vi "Oracle Popup.vi"(8 "error in":errorcluster, 11 "SR List in":T1[](array[typedef]) {"Last Updated" format="%<%x>T"}) -> (0 "error out":errorcluster, 1 "New SRs?":bool, 3 "SR List out":T1[](array[typedef]) {"Last Updated" format="%<%x>T"})   [LabVIEW 2018]
uses:
  SR Cluster.ctl
  <vilib>/Utility/miscctls.llb/LVPointTypeDef.ctl
  <vilib>/Utility/miscctls.llb/LVRectTypeDef.ctl
panel:
  in  "Ok Button":bool
  in  "Copied Text":string
  in  "Stop":bool
  # "In your Universal Work Queue in Oracle, right-click anywhere in the table and select \"Copy All Rows.\" Paste the copied information in the string container below, then press \"OK\"."
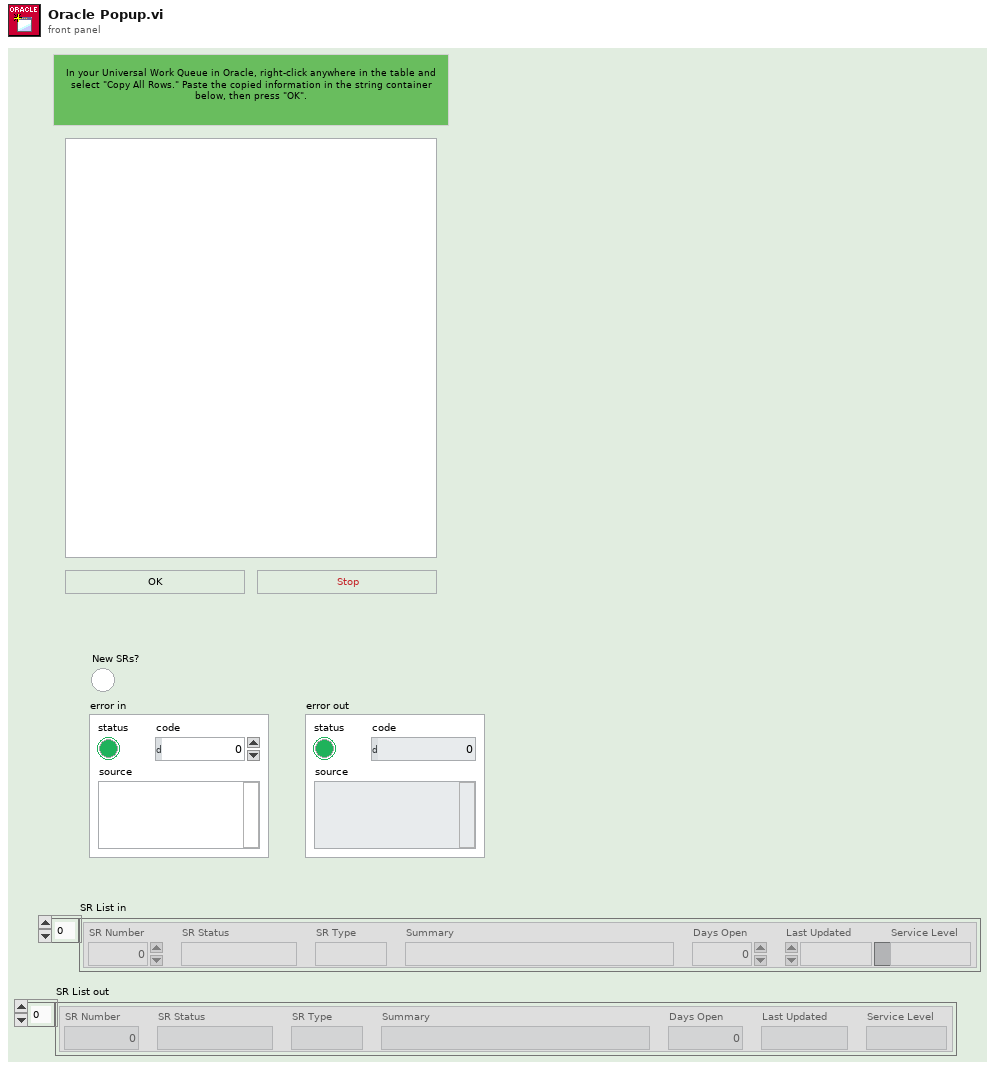
[diagram p1: front panel]
types:
  T1 = typedef "SR Cluster.ctl" = cluster{"SR Number":i32, "SR Status":string, "SR Type":string, "Summary":string, "Days Open":dbl, "Last Updated":timestamp, "Service Level":string}
  T2 = typedef "LVRectTypeDef.ctl" = cluster{"Left":i16, "Top":i16, "Right":i16, "Bottom":i16}
  T3 = typedef "LVPointTypeDef.ctl" = cluster{"Horizontal":i16, "Vertical":i16}
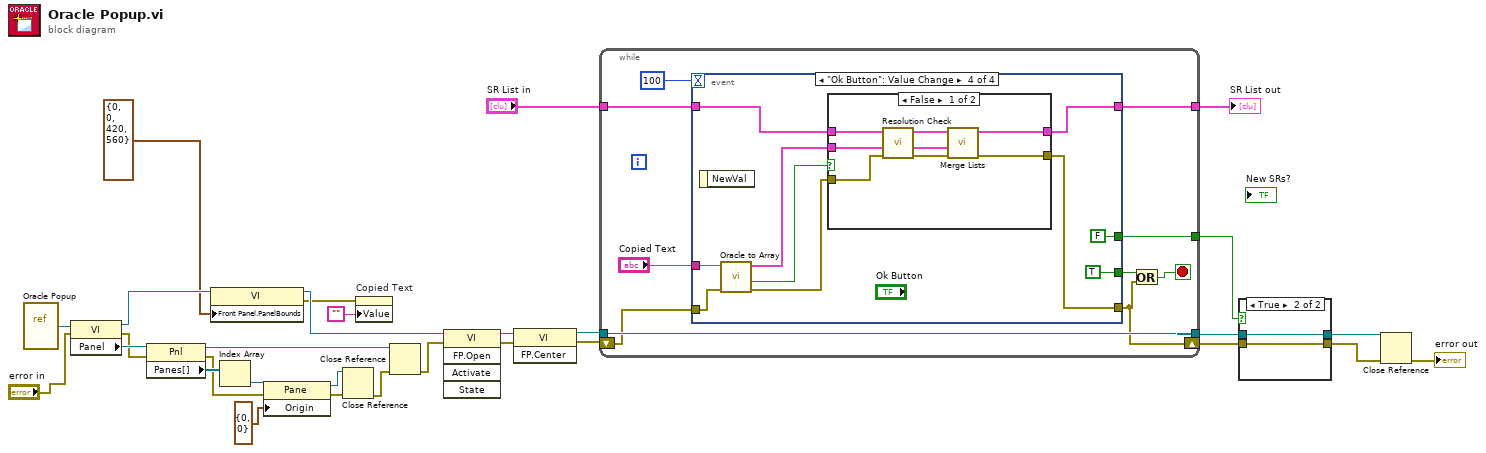
[diagram p0: block diagram]
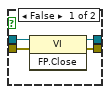
[diagram p2: hidden frame]
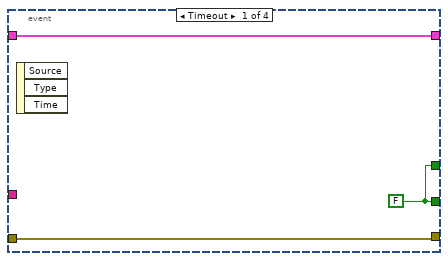
[diagram p3: hidden frame]
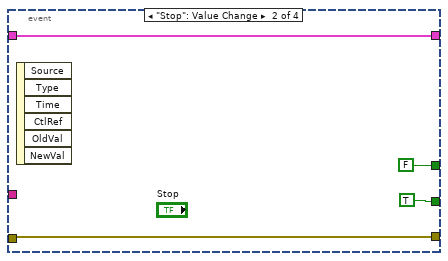
[diagram p4: hidden frame]
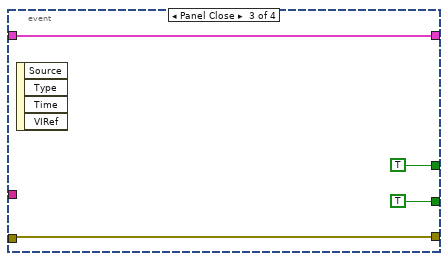
[diagram p5: hidden frame]
diagram:
  n1 = vi-ref "Oracle Popup.vi"() -> (w26:refnum<vi>)
  n2 = property class="VI"(reference=w26, error in="error in") -> (reference out=w11:refnum<vi>, error out=w16:errorcluster, "Panel"=w17:refnum<vi>)
  n3 = property class="Pnl"(reference=w17, error in=w16) -> (reference out=w18:refnum<vi>, error out=w23:errorcluster, "Panes[]"=w25:refnum<vi>[])
  n4 = property class="VI"(reference=w11, "Front Panel.PanelBounds"=T2 {"Left"=0, "Top"=0, "Right"=420, "Bottom"=560} ("Front Panel Window:Panel Bounds")) -> (reference out=w4:refnum<vi>, error out=w2:errorcluster)  [unwired: 1 in]
  n5 = Index Array(array=w25) -> (element=w24:refnum<vi>)  [unwired: 1 in]
  n6 = property class="Pane"(reference=w24, error in=w23, "Origin"=T3 {"Horizontal"=0, "Vertical"=0}) -> (reference out=w21:refnum<vi>, error out=w20:errorcluster)
  n7 = Close Reference(reference=w21, error in (no error)=w20) -> (error out=w19:errorcluster)
  n8 = property on="Copied Text" class="Str"(error in=w2, "Value"="") -> ()  [unwired: 1 in, 2 out]
  n9 = Close Reference(reference=w18, error in (no error)=w19) -> (error out=w5:errorcluster)
  n10 = invoke class="VI" method="FP.Open"(reference=w4, error in=w5) -> (reference out=w9:refnum<vi>, error out=w8:errorcluster)  [unwired: 3 in, 3 out]
  n11 = invoke class="VI" method="FP.Center"(reference=w9, error in=w8) -> (reference out=w6:refnum<vi>, error out=w7:errorcluster)  [unwired: 1 in, 1 out]
  n12 = while {
    tunnel: [w40] -> w30
    tunnel: w6 -> [w40]
    tunnel: [w38] -> w15
    tunnel: "SR List in" -> [w37]
    shift-right: [w32] -> w29
    shift-left: w7 -> [w35]
    tunnel: [w31] -> w1
    stop <- w33 stop-if-true
    n13 = event shown="[3] \"Ok Button\": Value Change" {
      selector: _ -> [_ _ _ _]
      dyn-events: _ -> [_ _ _ _]
      timeout: 100 -> [_ _ _ _]
      tunnel: [w41 TRUE ("Stop") TRUE ("Stop") TRUE ("Stop")] -> w34
      tunnel: [w43 w46 w51 w56] -> w38
      tunnel: w37 -> [w43 w46 w51 w57]
      tunnel: "Copied Text" -> [_ _ _ w60]
      tunnel: w35 -> [w42 w45 w49 w59]
      tunnel: [w42 w45 w49 w54] -> w32
      tunnel: [w41 FALSE ("Stop") TRUE ("Stop") FALSE ("Stop")] -> w31
      event Timeout {
        w41 = FALSE ("Stop")
        n14 = event-data() -> ()  [unwired: 1 in, 3 out]
      }
      event "Stop": Value Change {
        n15 = event-data() -> ()  [unwired: 1 in, 6 out]
      }
      event Panel Close {
        n16 = event-data() -> ()  [unwired: 1 in, 4 out]
      }
      event "Ok Button": Value Change {
        n17 = event-data() -> ()  [unwired: 1 in, 1 out]
        n18 = call "Oracle to Array.vi"("error in"=w59, "string in"=w60) -> ("error out"=w53:errorcluster, "Empty?"=w58:bool, "list out"=w55:T1[])  [unwired: 7 in]
        n19 = case shown="False" w58 {
          tunnel: w57 -> [w69 w71]
          tunnel: [w66 w71] -> w56
          tunnel: w55 -> [w68 _]
          tunnel: [w64 w70] -> w54
          tunnel: w53 -> [w67 w70]
          frame False {
            n20 = call "Resolution Check.vi"("error in"=w67, "new list in"=w68, "SR List in"=w69) -> ("error out"=w63:errorcluster, "new list out"=w62:T1[], "list out"=w65:T1[])  [unwired: 6 in]
            n21 = call "Merge Lists.vi"("error in"=w63, "new list in"=w62, "list in"=w65) -> ("error out"=w64:errorcluster, "list out"=w66:T1[])  [unwired: 7 in]
          }
          frame True {
          }
        }
      }
    }
    n22 = Or(x=w34, y=w32) -> (x .or. y?=w33:bool)
  }
  "SR List out" <- w15
  n23 = case shown="True" w1 {
    tunnel: w30 -> [w75 w77]
    tunnel: w29 -> [w74 w76]
    tunnel: [w73 w77] -> w28
    tunnel: [w72 w76] -> w27
    frame False {
      n24 = invoke class="VI" method="FP.Close"(reference=w75, error in=w74) -> (reference out=w73:refnum<vi>, error out=w72:errorcluster)  [unwired: 1 in, 1 out]
    }
    frame True {
    }
  }
  n25 = Close Reference(reference=w28, error in (no error)=w27) -> (error out=→"error out":errorcluster)
